vi "OAT Single Stage Decimation.vi"(7 "reset? (True)":bool=TRUE, 8 "error in (no error)":errorcluster, 9 "filter":T1={"coefficients"=[], "factor"=1} {"coefficients" format="%.2f"}, 11 "X":dbl[](array[numeric]) format="%.2f") -> (0 "error out":errorcluster, 3 "Y":dbl[](array[numeric]) format="%.2f")   [LabVIEW 2017, in "SoundVib_Resampling.lvlib"]
doc: "Decimate the input sequence <B>X</B> with the single stage decimation filter specified by <B>filter</B>."
uses:
  <vilib>/addons/Sound and Vibration/Order Analysis/Resample Order Tracking/SoundVib_Resampling.lvlib
  <vilib>/addons/_NISVFA/_Shared subVIs/Controls/OAT Decimation Filter.ctl
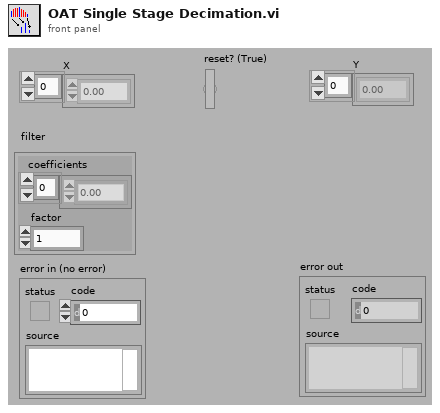
[diagram p1: front panel]
types:
  T1 = typedef "OAT Decimation Filter.ctl" = cluster{"coefficients":dbl[], "factor":i32}
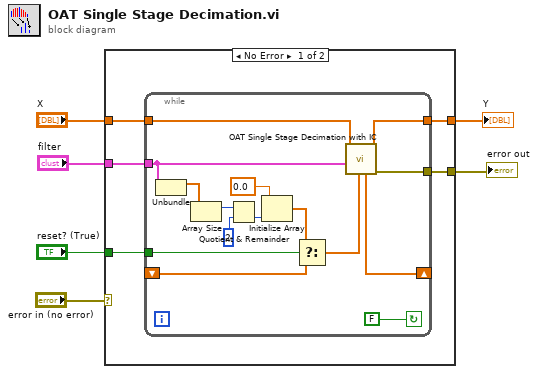
[diagram p0: block diagram]
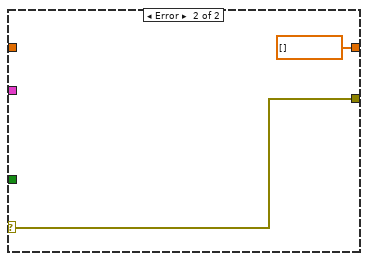
[diagram p2: hidden frame]
diagram:
  n1 = case shown="No Error" "error in (no error)" {
    selector: "error in (no error)" -> [_ w28]
    tunnel: "filter" -> [w11 _]
    tunnel: [w10 dbl[] [] ("Y")] -> w5
    tunnel: "X" -> [w9 _]
    tunnel: "reset? (True)" -> [w8 _]
    tunnel: [w7 w28] -> w2
    frame No Error {
      n2 = while {
        tunnel: w8 -> [w22]
        shift-left: _ -> [w21]
        shift-right: [w24] -> _
        tunnel: w9 -> [w25]
        tunnel: [w26] -> w10
        tunnel: w11 -> [w13]
        tunnel: [w12] -> w7
        stop <- FALSE continue-if-true
        n3 = Unbundle(w13) -> ("coefficients"=w14:dbl[])  [unwired: 1 out]
        n4 = Array Size(array=w14) -> (size(s)=w17:i32)
        n5 = Quotient & Remainder(x=w17, y=2) -> (floor(x/y)=w18:i32)  [unwired: 1 out]
        n6 = Initialize Array(0.0 ("Element Data"), w18) -> (w19:dbl[])
        n7 = Select(t=w19, s=w22, f=w21) -> (s? t:f=w20:dbl[])
        n8 = call <vilib>:"OAT Single Stage Decimation with IC.vi"("initial state"=w20, "filter"=w13, "X"=w25) -> ("error out"=w12:errorcluster, "Y"=w26:dbl[], "final state"=w24:dbl[])  [unwired: 6 in]
      }
    }
    frame Error {
    }
  }
  "Y" <- w5
  "error out" <- w2
